vi "Read UserPwd DB Obj.vi"(11 "VacuumLines in":refnum<class "VacuumLines.lvclass">) -> (2 "UserPwd DB.lvlib:UserPwd DB.lvclass":refnum<class "UserPwd DB.lvclass">, 3 "VacuumLines out":refnum<class "VacuumLines.lvclass">)   [LabVIEW 2016, in "Hardware.lvlib" / "VacuumLine.lvlib" / "VacuumLines.lvclass"]
uses:
  <userlib>/Common Components/Hardware/Abstract System/VacuumLine/VacuumLines/VacuumLines.lvclass
  <userlib>/Common Components/UserPwd DB/UserPwd DB/UserPwd DB.lvclass
  <userlib>/Common Components/Hardware/Abstract System/VacuumLine/VacuumLines/VacuumLines.lvclass/VacuumLines.ctl
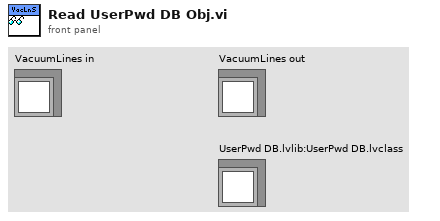
[diagram p1: front panel]
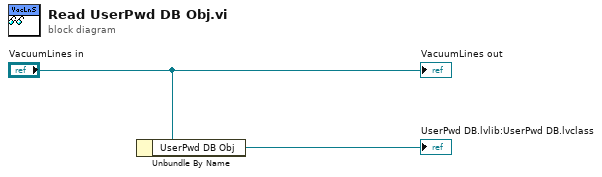
[diagram p0: block diagram]
diagram:
  n1 = Unbundle By Name("VacuumLines in") -> ("UserPwd DB Obj"=→"UserPwd DB.lvlib:UserPwd DB.lvclass":refnum<class "UserPwd DB.lvclass">)
  "VacuumLines out" <- "VacuumLines in"
